vi "SampleGetPositionAllSlaves.vi"() -> ()   [LabVIEW 2009]
panel:
  out "Output:":string
  out "DeviceKey List Out":string[](array[string])
  out "error out":errorcluster
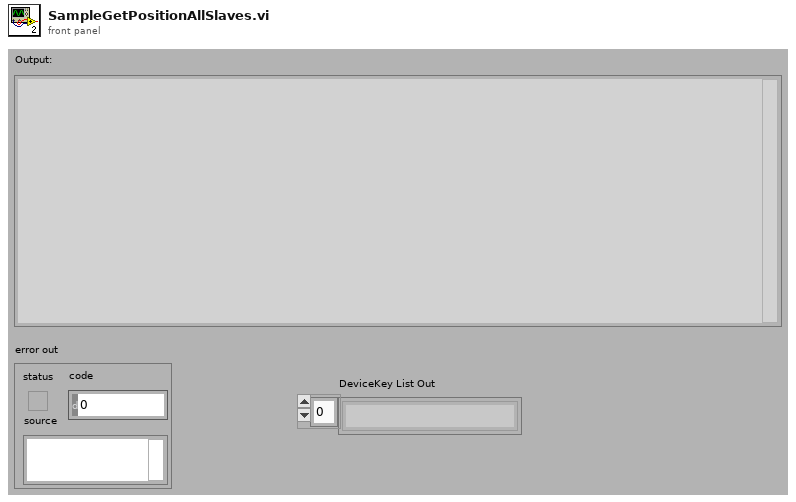
[diagram p1: front panel]
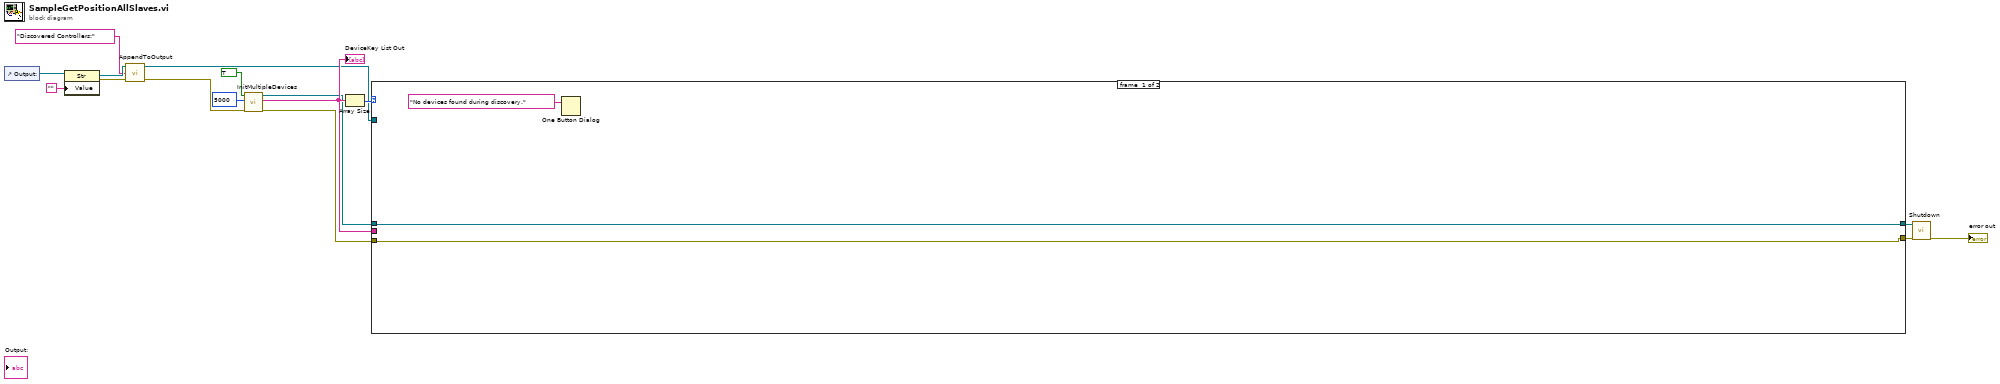
[diagram p0: block diagram]
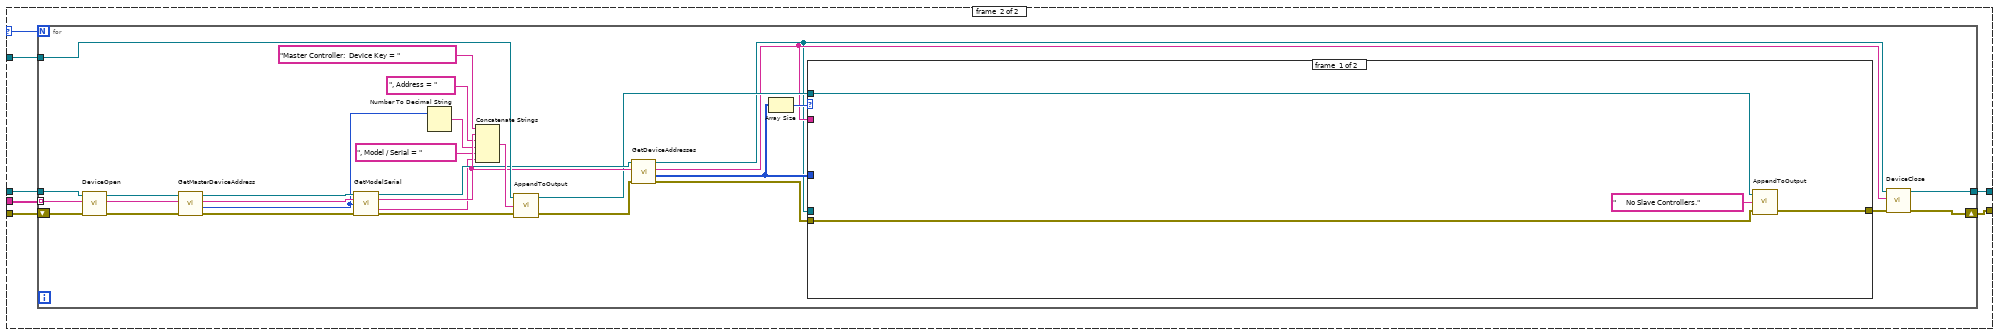
[diagram p2: hidden frame]
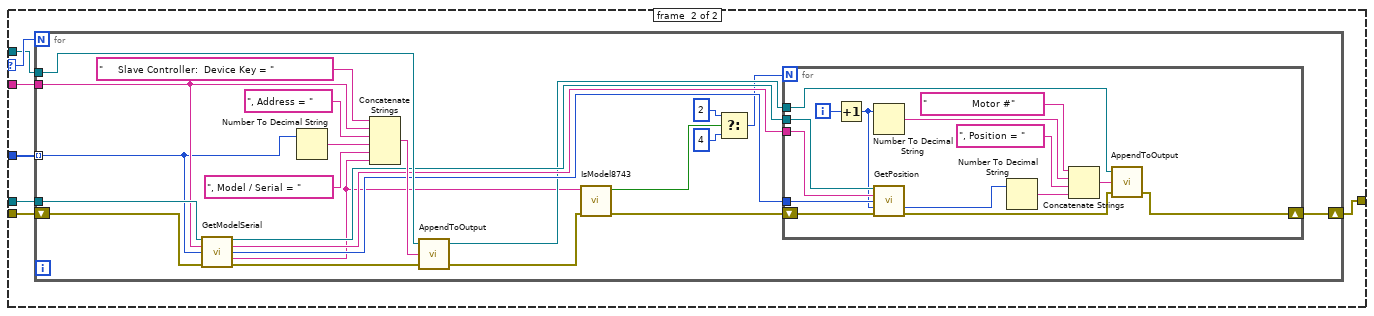
[diagram p3: hidden frame]
diagram:
  n1 = control-ref of="Output:"() -> (w7:refnum<vi>)
  n2 = property class="Str"(reference=w7, "Value"="") -> (reference out=w5:refnum<vi>, error out=w4:errorcluster)  [unwired: 1 in]
  n3 = call "AppendToOutput.vi"("error in"=w4, "Input String"="Discovered Controllers:", "Output Refnum In"=w5) -> ("error out"=w3:errorcluster, "Output Refnum Out"=w1:refnum<vi>)  [unwired: 1 in]
  n4 = call "InitMultipleDevices.vi"("error in (no error)"=w3, "msecDelayForDiscovery"=5000, "logging"=TRUE) -> ("error out"=w10:errorcluster, "DeviceKey List Out"=w12:string[], "CmdLib Out"=w11:refnum<k24>)  [unwired: 2 in]
  "DeviceKey List Out" <- w12
  n5 = Array Size(array=w12) -> (size(s)=w13:i32)
  n6 = case shown="1, Default" w13 {
    selector: w13 -> [_ w26]
    tunnel: w12 -> [_ w25]
    tunnel: w11 -> [w18 w24]
    tunnel: w10 -> [w19 w23]
    tunnel: [w19 w20] -> w9
    tunnel: [w18 w22] -> w8
    tunnel: w1 -> [_ w21]
    frame #0 {
      n7 = One Button Dialog(message="No devices found during discovery.") -> ()  [unwired: 1 in, 1 out]
    }
    frame #1 {
      n8 = for {
        N: w26 -> [_]
        tunnel: w25 -> [w54] mode=indexing
        tunnel: w24 -> [w56]
        tunnel: [w55] -> w22
        tunnel: w21 -> [w52]
        shift-right: [w27] -> w20
        shift-left: w23 -> [w53]
        n9 = call "DeviceOpen.vi"("error in (no error)"=w53, "DeviceKey In"=w54, "CmdLib In"=w56) -> ("error out"=w46:errorcluster, "DeviceKey Out"=w47:string, "CmdLib Out"=w48:refnum<k24>)  [unwired: 2 in]
        n10 = call "GetMasterDeviceAddress.vi"("error in (no error)"=w46, "DeviceKey In"=w47, "CmdLib In"=w48) -> ("error out"=w43:errorcluster, "Device Address"=w28:i32, "DeviceKey Out"=w42:string, "CmdLib Out"=w41:refnum<k24>)  [unwired: 1 in]
        n11 = call "GetModelSerial.vi"("CmdLib In"=w41, "DeviceKey In"=w42, "Device Address In"=w28, "error in (no error)"=w43) -> ("CmdLib Out"=w44:refnum<k24>, "DeviceKey Out"=w40:string, "Model / Serial"=w36:string, "error out"=w45:errorcluster)  [unwired: 7 in, 1 out]
        n12 = Number To Decimal String(number=w28) -> (decimal integer string=w38:string)  [unwired: 1 in]
        n13 = Concatenate Strings("Master Controller:  Device Key = " ("string"), w40, ", Address = " ("string"), w38, ", Model / Serial = " ("string"), w36) -> (w51:string)
        n14 = call "AppendToOutput.vi"("error in"=w45, "Input String"=w51, "Output Refnum In"=w52) -> ("error out"=w49:errorcluster, "Output Refnum Out"=w34:refnum<vi>)  [unwired: 1 in]
        n15 = call "GetDeviceAddresses.vi"("error in (no error)"=w49, "DeviceKey In"=w40, "CmdLib In"=w44) -> ("error out"=w33:errorcluster, "Device Addresses"=w31:i32[], "DeviceKey Out"=w30:string, "CmdLib Out"=w29:refnum<k24>)  [unwired: 1 in]
        n16 = Array Size(array=w31) -> (size(s)=w35:i32)
        n17 = case shown="1, Default" w35 {
          selector: w35 -> [_ w67]
          tunnel: w34 -> [w59 w63]
          tunnel: w33 -> [w58 w61]
          tunnel: [w57 w64] -> w32
          tunnel: w31 -> [_ w66]
          tunnel: w30 -> [_ w65]
          tunnel: w29 -> [_ w62]
          frame #0 {
            n18 = call "AppendToOutput.vi"("error in"=w58, "Input String"="     No Slave Controllers.", "Output Refnum In"=w59) -> ("error out"=w57:errorcluster)  [unwired: 1 in, 1 out]
          }
          frame #1 {
            n19 = for {
              N: w67 -> [_]
              tunnel: w66 -> [w82] mode=indexing
              tunnel: w65 -> [w83]
              tunnel: w63 -> [w86]
              tunnel: w62 -> [w84]
              shift-right: [w78] -> w64
              shift-left: w61 -> [w81]
              n20 = call "GetModelSerial.vi"("CmdLib In"=w84, "DeviceKey In"=w83, "Device Address In"=w82, "error in (no error)"=w81) -> ("CmdLib Out"=w79:refnum<k24>, "DeviceKey Out"=w80:string, "Device Address Out"=w77:i32, "Model / Serial"=w70:string, "error out"=w75:errorcluster)  [unwired: 7 in]
              n21 = Number To Decimal String(number=w82) -> (decimal integer string=w88:string)  [unwired: 1 in]
              n22 = Concatenate Strings("     Slave Controller:  Device Key = " ("string"), w83, ", Address = " ("string"), w88, ", Model / Serial = " ("string"), w70) -> (w85:string)
              n23 = call "AppendToOutput.vi"("error in"=w75, "Input String"=w85, "Output Refnum In"=w86) -> ("error out"=w69:errorcluster, "Output Refnum Out"=w76:refnum<vi>)  [unwired: 1 in]
              n24 = call "IsModel8743.vi"("error in"=w69, "Model / Serial"=w70) -> ("error out"=w68:errorcluster, "Boolean"=w74:bool)  [unwired: 8 in]
              n25 = Select(t=2, s=w74, f=4) -> (s? t:f=w71:i32)
              n26 = for {
                N: w71 -> [_]
                tunnel: w80 -> [w105]
                tunnel: w79 -> [w104]
                tunnel: w77 -> [w102]
                tunnel: w76 -> [w100]
                shift-right: [w101] -> w78
                shift-left: w68 -> [w103]
                i -> [w96]
                n27 = Increment(x=w96) -> (x+1=w92:i32)
                n28 = Number To Decimal String(number=w92) -> (decimal integer string=w97:string)  [unwired: 1 in]
                n29 = call "GetPosition.vi"("CmdLib In"=w104, "DeviceKey In"=w105, "Device Address In"=w102, "Motor"=w92, "error in (no error)"=w103) -> ("Position"=w95:i32, "error out"=w91:errorcluster)  [unwired: 6 in, 3 out]
                n30 = Number To Decimal String(number=w95) -> (decimal integer string=w94:string)  [unwired: 1 in]
                n31 = Concatenate Strings("               Motor #" ("Input String"), w97, ", Position = " ("string"), w94) -> (w98:string)
                n32 = call "AppendToOutput.vi"("error in"=w91, "Input String"=w98, "Output Refnum In"=w100) -> ("error out"=w101:errorcluster)  [unwired: 1 in, 1 out]
              }
            }
          }
        }
        n33 = call "DeviceClose.vi"("error in (no error)"=w32, "DeviceKey In"=w30, "CmdLib In"=w29) -> ("error out"=w27:errorcluster, "CmdLib Out"=w55:refnum<k24>)  [unwired: 2 in, 1 out]
      }
    }
  }
  n34 = call "Shutdown.vi"("error in (no error)"=w9, "CmdLib In"=w8) -> ("error out"=→"error out":errorcluster)  [unwired: 4 in, 1 out]
